vi "Write State to Info.vi"(7 "Write to Terminal":bool=TRUE, 8 "error in (no error)":errorcluster, 9 "gRPC Port":i32, 10 "Command":T1, 11 "Plugin Name":string) -> (0 "error out":errorcluster)   [LabVIEW 2021, in "CIFLogs.lvlib"]
uses:
  CIFLogs.lvlib
  Typedef/Message Type.ctl
  Typedef/Plugin State Commands.ctl
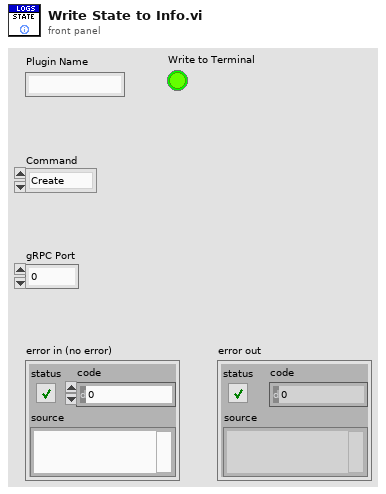
[diagram p1: front panel]
types:
  T1 = typedef "CIFLogs.lvlib/Plugin State Commands.ctl" = enum16{"Create", "Configure", "Run", "Pause", "Destroy"}
  T2 = typedef "CIFLogs.lvlib/Message Type.ctl" = enum16{"Error", "Information", "Print Terminal", "Configuration"}
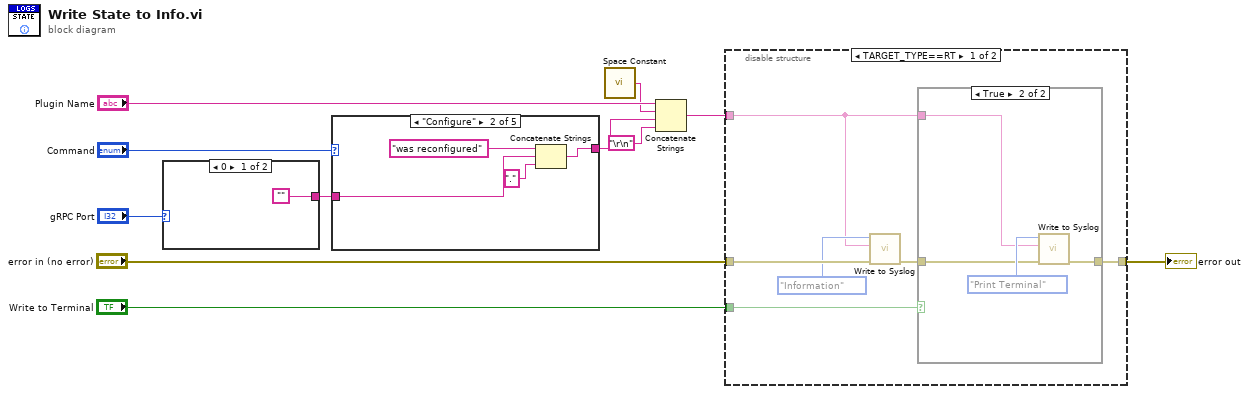
[diagram p0: block diagram]
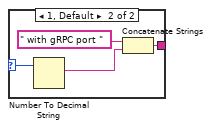
[diagram p2: hidden frame]
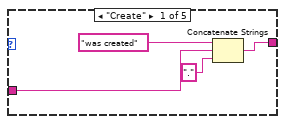
[diagram p3: hidden frame]
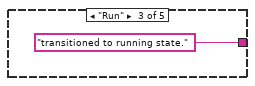
[diagram p4: hidden frame]
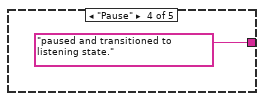
[diagram p5: hidden frame]
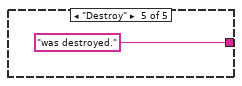
[diagram p6: hidden frame]
diagram:
  n1 = case shown="0" "gRPC Port" {
    selector: "gRPC Port" -> [_ w16]
    tunnel: ["" w13] -> w2
    frame 0 {
    }
    frame 1, Default {
      n2 = Number To Decimal String(number=w16) -> (decimal integer string=w14:string)  [unwired: 1 in]
      n3 = Concatenate Strings(" with gRPC port ", w14) -> (w13:string)
    }
  }
  n4 = case shown="\"Configure\"" "Command" {
    tunnel: [w17 w21 "transitioned to running state." "paused and transitioned to listening state." "was destroyed."] -> w6
    tunnel: w2 -> [w19 w23 _ _ _]
    frame "Create" {
      n5 = Concatenate Strings("was created", w19, ".") -> (w17:string)
    }
    frame "Configure" {
      n6 = Concatenate Strings("was reconfigured", w23, ".") -> (w21:string)
    }
    frame "Run" {
    }
    frame "Pause" {
    }
    frame "Destroy" {
    }
  }
  n7 = call <vilib>:"Space Constant.vi"() -> ("String"=w5:string)
  n8 = Concatenate Strings("Plugin Name", w5, w6, "\r\n") -> (w8:string)
  n9 = disable-structure shown="TARGET_TYPE==RT" {
    disable-tunnel: "error in (no error)" -> [w32 _]
    disable-tunnel: [w33 _] -> w10
    disable-tunnel: w8 -> [w29 _]
    disable-tunnel: "Write to Terminal" -> [w28 _]
    frame condition #0 {
      n10 = call "Write to Syslog.vi"("error in (no error)"=w32, "message"=w29, "CIF Message Type"=Message_Type."Information") -> ("error out"=w31:errorcluster)  [unwired: 8 in]
      n11 = case shown="True" w28 {
        tunnel: [w34 w38] -> w33
        tunnel: w31 -> [w34 w36]
        tunnel: w29 -> [_ w35]
        frame False {
        }
        frame True {
          n12 = call "Write to Syslog.vi"("error in (no error)"=w36, "message"=w35, "CIF Message Type"=Message_Type."Print Terminal") -> ("error out"=w38:errorcluster)  [unwired: 8 in]
        }
      }
    }
    frame condition #1 (active) {
    }
  }
  "error out" <- w10
